vi "ADMIN -Process Customize for Company.vi"(0 "SET":T2=enum."GET ALL", 2 "CfgValues":string[][](array[string])=[["", ""], ["CompanyName", "ABC Test Labs Inc"], ["LogoFileName", "ABC.png"], ["CSACategory", "II"], ["HomeAddrLine00", "McIntosh Lalani Engineering LTD."], ["HomeAddrLine01", "Bay 10,4604 - 13th Street NE"], ["HomeAddLine02", "Calgary AB  T2E 6P1"], ["HomeAddrLine03", "CANADA"], ["", ""], ["DeltaTestTime", "120"], ["", ""], ["PDFRptDir", "C:\\Program Files (x86)\\BreakTest\\PDF_ARCHIVE"], ["PDFRes", "8-Bit Gray Scale"], ["PDFDrvName", "Black Ice PDF"], ["PDFAlertDays", "2"], ["WebPortalURL", "-"], ["", ""], ["DshBrdEnabled", "Yes"], ["DshBrdEvntNeedsAction", "Yes"], ["DshBrdEvntNew", "Yes"], ["DshBrdEvntUpdate", "Yes"], ["DshBrdEvntSignature", "Yes"], ["DshBrdEvntAgeData", "Yes"], ["", ""], ["EmailSvrAddr", "shawmail.cg.shawcable.net"], ["EmailAddr", "emmanual@shaw.ca"], ["EmailAccName", "Immanuel Nwachukwu"], ["EmailSize", "5"], ["", ""], ["FTPDir", "-"], ["FTPAddr", "ftp.mezintel.com"], ["FTPUser", "breaktestrpts@mezintel.com"], ["FTPPswd", "Break123"], ["", ""], ["UtilStartDate", "2011/09/26"], ["GSTPercent", "5"], ["CostPerTest", "1.5"], ["VendorAddrLine00", "Mezintel Inc."], ["VendorAddrLine01", "20 Citadel Hills Green NW"], ["VendorAddrLine02", "Calgary, AB, T3G 3T5"], ["VendorAddrLine03", "CANADA"]], 3 "KEY":string, 5 "error in (no error)":errorcluster, 8 "path to PNG file":path) -> (13 "Found":bool, 14 "ALL -Out":T1={"CurrPath"=path "C:/MEZINTEL PROJECTS/PERFORCE MEZINTEL PROJECTS/BreakTest 3/BreakTest Source/SOURCE CODE", "LogoPic"=bytes[30000], "LogoPicRed"=bytes[2727], "CoName"="ABC Test Labs Inc", "CSACategory"="II", "Home CoID|DivID"=["47", "52"], "ParmKey|Value"=[["LogoFileName", "ABC.png"], ["CompanyName", "ABC Test Labs Inc"], ["CSACategory", "II"], ["PDFRptDir", "C:\\Program Files (x86)\\BreakTest\\PDF_ARCHIVE"], ["PDFRes", "8-Bit Gray Scale"], ["DshBrdEnabled", "Yes"], ["EmailSvrAddr", "shawmail.cg.shawcable.net"], ["EmailAddr", "emmanual@shaw.ca"], ["EmailAccName", "Immanuel Nwachukwu"], ["EmailSize", "5"], ["PDFDrvName", "Black Ice PDF"], ["PDFAlertDays", "2"], ["FTPAddr", "ftp.mezintel.com"], ["FTPUser", "breaktestrpts@mezintel.com"], ["FTPPswd", "Break123"], ["WebPortalURL", "-"]], "PicRef"=refnum, "DBParmKey|Value"=[]}, 15 "VALUE":string, 18 "ClrRes":i32, 19 "error out":errorcluster)   [LabVIEW 2019]
uses:
  ctlFNCoCustomization.ctl
  ctlADMIN-CoCfgParamsOut.ctl
  <vilib>/Utility/config.llb/Read Key (String).vi
  <vilib>/Utility/config.llb/Write Key (String).vi
  <vilib>/Utility/config.llb/NI_LVConfig.lvlib
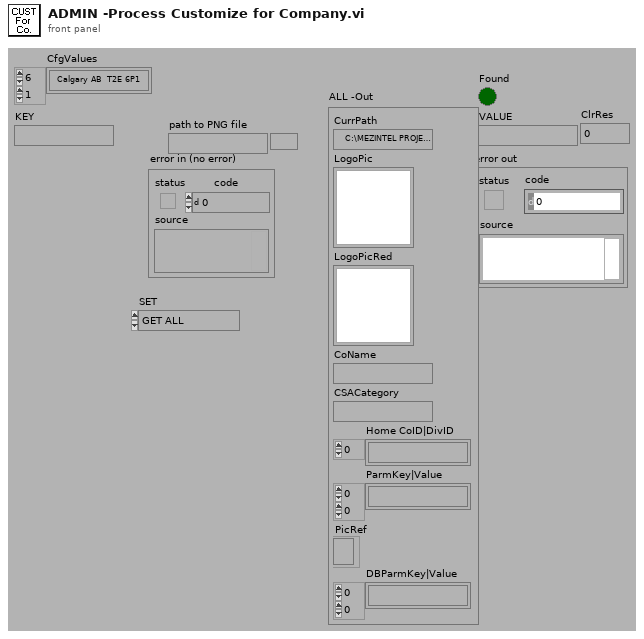
[diagram p1: front panel]
types:
  T1 = typedef "ctlADMIN-CoCfgParamsOut.ctl" = cluster{"CurrPath":path, "LogoPic":picture, "LogoPicRed":picture, "CoName":string, "CSACategory":string, "Home CoID|DivID":string[], "ParmKey|Value":string[][], "PicRef":refnum<k7>, "DBParmKey|Value":string[][]}
  T2 = typedef "ctlFNCoCustomization.ctl" = enum16{"pre-init", "Init", "Write Co. Info to ini", "GET CFG PARAM", "GET Param Value for Name", "GET ALL"}
  T3 = cluster{"path to PNG file":path, "LogoPic":picture, "LogoPicRed":picture, "CoName":string, "CSACategory":string, "Home CoID|DivID":string[], "ParmKey|Value":string[][], "PicRef":refnum<k7>, "DBParmKey|Value":string[][]}
  T4 = typedef "NI_LVConfig.lvlib/Config Data RefNum.ctl" = refnum<k1>
  T5 = typedef "imagedata.ctl" = cluster{"image type":i32, "image depth":i32, "image":u8[], "mask":u8[], "colors":u32[], "Rectangle":cluster{"left":i16, "top":i16, "right":i16, "bottom":i16}}
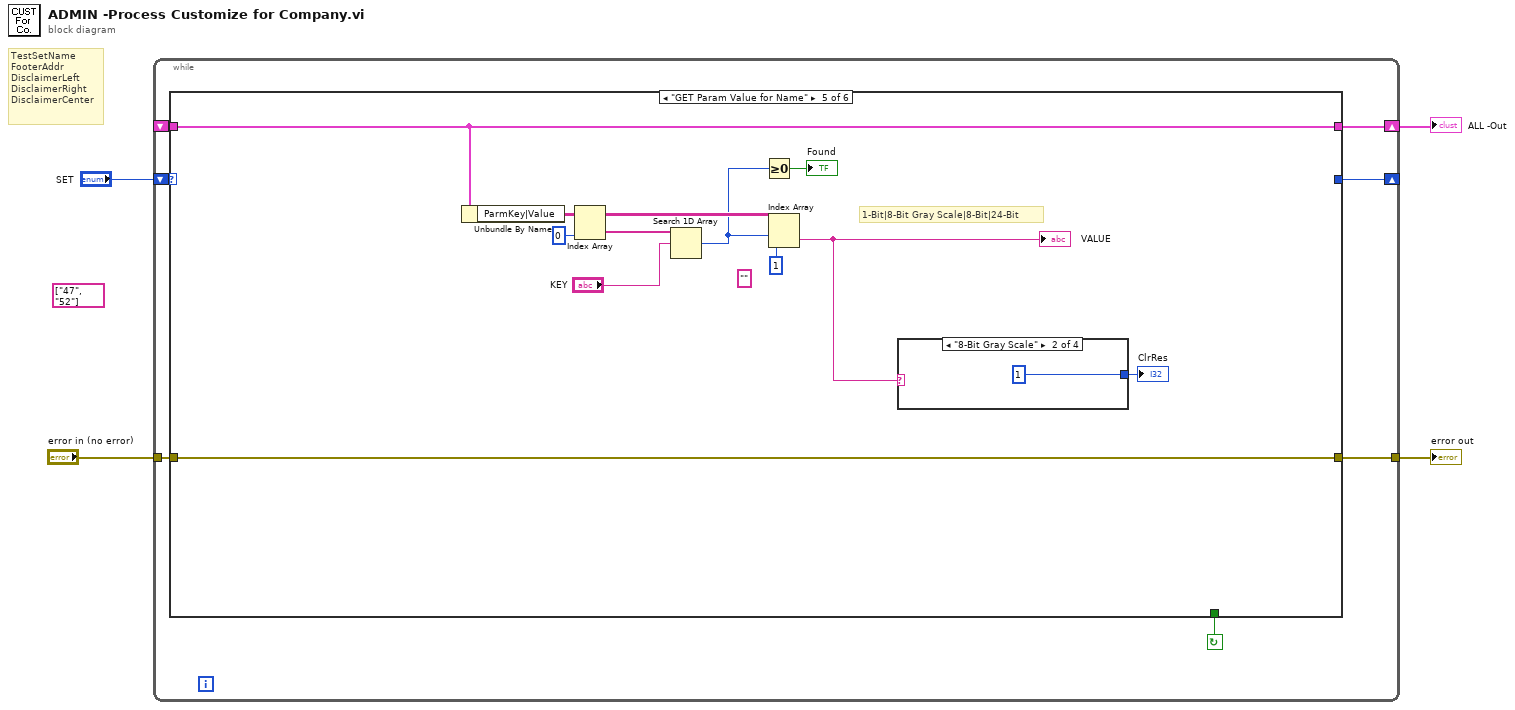
[diagram p0: block diagram]
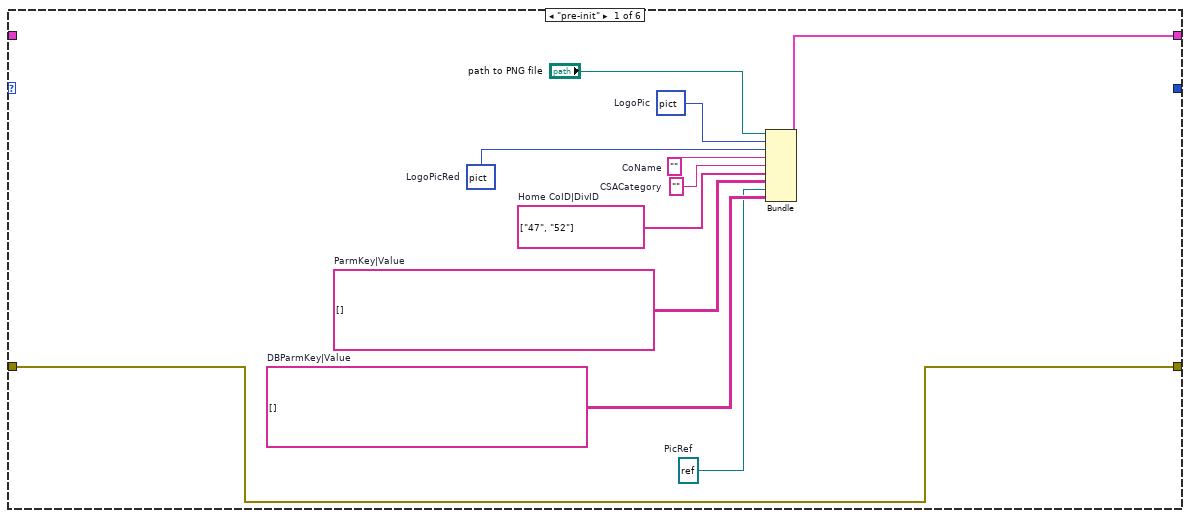
[diagram p2: hidden frame]
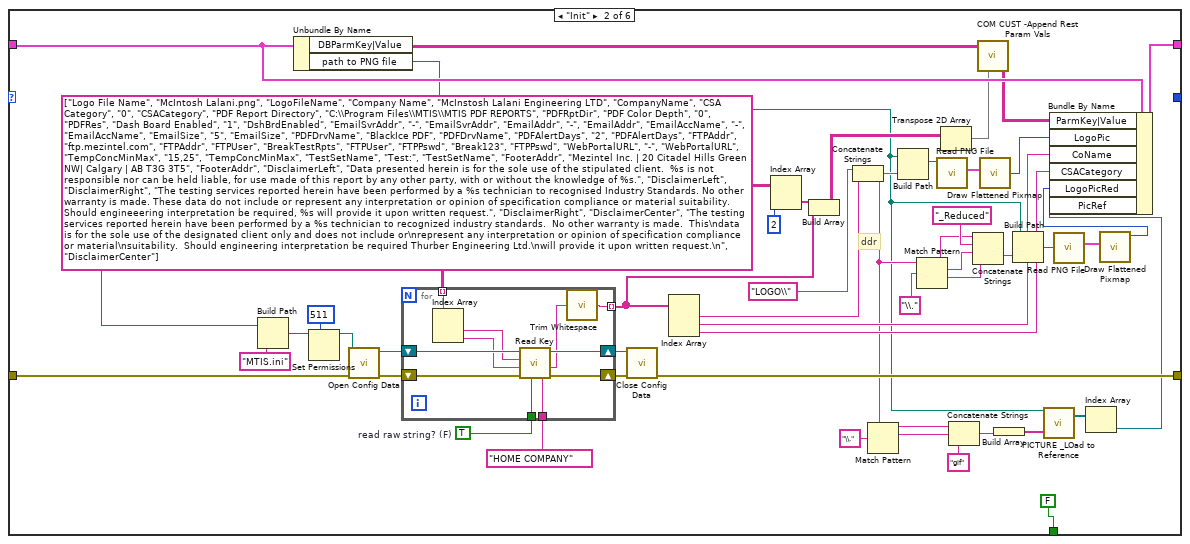
[diagram p3: hidden frame]
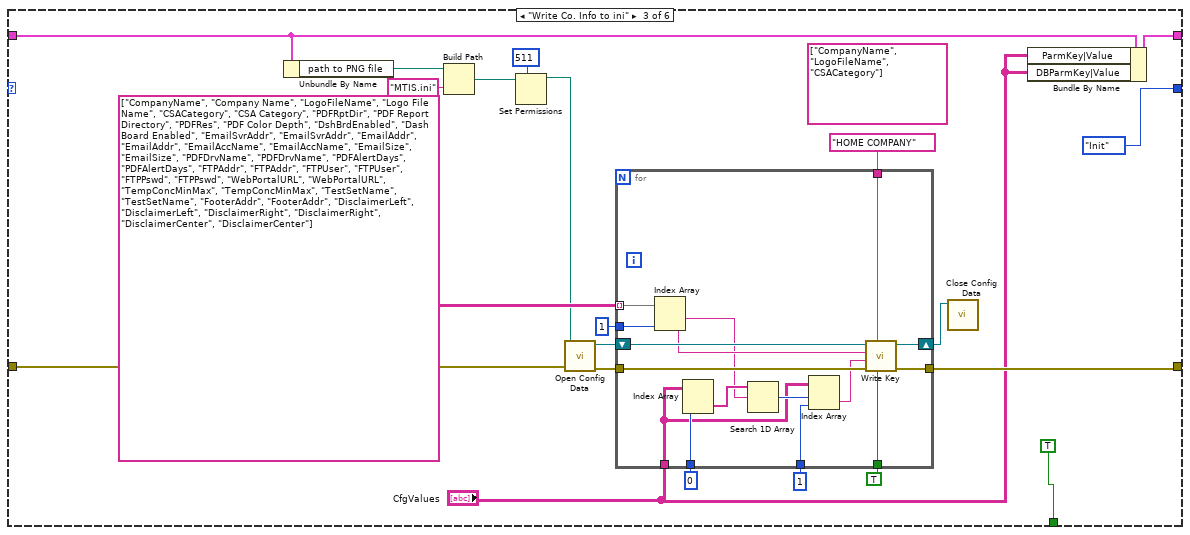
[diagram p4: hidden frame]
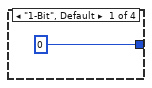
[diagram p6: hidden frame]
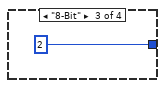
[diagram p7: hidden frame]
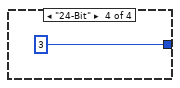
[diagram p8: hidden frame]
diagram:
  (unwired) string[] ["47", "52"] ("Home CoID|DivID")
  # "TestSetName\nFooterAddr\nDisclaimerLeft\nDisclaimerRight\nDisclaimerCenter"
  n1 = while {
    tunnel: [w10] -> w3
    tunnel: "error in (no error)" -> [w9]
    shift-right: [w6] -> w1
    shift-left: _ -> [w7]
    shift-right: [w5] -> _
    shift-left: "SET" -> [w11]
    stop <- w8 continue-if-true
    n2 = case shown="\"GET Param Value for Name\"" w11 {
      tunnel: [w13 w67 w84 w121 w132 w138] -> w10
      tunnel: w9 -> [w13 w66 w102 w121 w132 w138]
      tunnel: [_ FALSE TRUE _ _ _] -> w8
      tunnel: w7 -> [_ w52 w92 w120 w131 w137]
      tunnel: [w14 w57 w91 w120 w131 w137] -> w6
      tunnel: [_ _ ctlFNCoCustomization."Init" ("SET") _ _ _] -> w5
      frame "pre-init" {
        w22 = string[][] []  # DBParmKey|Value
        w21 = refnum<k7> refnum  # PicRef
        w20 = picture data[5B]  # LogoPicRed
        w19 = string[][] []  # ParmKey|Value
        w18 = string[] ["47", "52"]  # Home CoID|DivID
        w15 = picture data[5B]  # LogoPic
        w17 = ""  # CSACategory
        w16 = ""  # CoName
        n3 = Bundle("path to PNG file"="path to PNG file", "LogoPic"=w15, "LogoPicRed"=w20, "CoName"=w16, "CSACategory"=w17, "Home CoID|DivID"=w18, "ParmKey|Value"=w19, "PicRef"=w21, "DBParmKey|Value"=w22) -> (w14:T3)  [unwired: 1 out]
      }
      frame "Init" {
        w33 = string[][] [["Logo File Name", "McIntosh Lalani.png", "LogoFileName"], ["Company Name", "McInstosh Lalani Engineering LTD", "CompanyName"], ["CSA Category", "0", "CSACategory"], ["PDF Report Directory", "C:\\Program Files\\MTIS\\MTIS PDF REPORTS", "PDFRptDir"], ["PDF Color Depth", "0", "PDFRes"], ["Dash Board Enabled", "1", "DshBrdEnabled"], ["EmailSvrAddr", "-", "EmailSvrAddr"], ["EmailAddr", "-", "EmailAddr"], ["EmailAccName", "-", "EmailAccName"], ["EmailSize", "5", "EmailSize"], ["PDFDrvName", "BlackIce PDF", "PDFDrvName"], ["PDFAlertDays", "2", "PDFAlertDays"], ["FTPAddr", "ftp.mezintel.com", "FTPAddr"], ["FTPUser", "BreakTestRpts", "FTPUser"], ["FTPPswd", "Break123", "FTPPswd"], ["WebPortalURL", "-", "WebPortalURL"], ["TempConcMinMax", "15,25", "TempConcMinMax"], ["TestSetName", "Test:", "TestSetName"], ["FooterAddr", "Mezintel Inc. | 20 Citadel Hills Green NW| Calgary | AB T3G 3T5", "FooterAddr"], ["DisclaimerLeft", "Data presented herein is for the sole use of the stipulated client.  %s is not responsible nor can be held liable, for use made of this report by any other party, with or without the knowledge of %s.", "DisclaimerLeft"], ["DisclaimerRight", "The testing services reported herein have been performed by a %s technician to recognised Industry Standards. No other warranty is made. These data do not include or represent any interpretation or opinion of specification compliance or material suitability. Should engineeering interpretation be required, %s will provide it upon written request.", "DisclaimerRight"], ["DisclaimerCenter", "The testing services reported herein have been performed by a %s technician to recognized industry standards.  No other warranty is made.  This\ndata is for the sole use of the designated client only and does not include or\nrepresent any interpretation or opinion of specification compliance or material\nsuitability.  Should engineering interpretation be required Thurber Engineering Ltd.\nwill provide it upon written request.\n", "DisclaimerCenter"]]
        w61 = TRUE  # read raw string? (F)
        # "ddr"
        n4 = Unbundle By Name(w52) -> ("DBParmKey|Value"=w26:string[][], "path to PNG file"=w23:path)
        n5 = Build Path(base path=w23, name or relative path="MTIS.ini") -> (appended path=w63:path)
        n6 = Set Permissions(7:i16 511 ("permissions"), 11:w63) -> (3:w28:path)  [unwired: 1 in, 3 out]
        n7 = call <vilib>:"Open Config Data.vi"("error in (no error)"=w66, "configuration file path"=w28) -> ("error out"=w65:errorcluster, "refnum"=w62:T4)  [unwired: 7 in, 1 out]
        n8 = for {
          shift-right: [w79] -> w60
          shift-left: w62 -> [w80]
          tunnel: w33 -> [w78] mode=indexing
          tunnel: w61 -> [w75]
          shift-right: [w81] -> w64
          shift-left: w65 -> [w82]
          tunnel: [w72] -> w29 mode=indexing
          tunnel: "HOME COMPANY" ("section") -> [w73]
          n9 = Index Array(array=w78) -> (element #1=w77:string, element #2=w76:string)  [unwired: 2 in]
          n10 = call-poly <vilib>:"Read Key.vi"("read raw string? (F)"=w75, "section"=w73, "error in (no error)"=w82, "default value"=w76, "key"=w77, "refnum"=w80) -> ("error out"=w81:errorcluster, "value"=w74:string, "refnum out"=w79:T4)  [unwired: 3 out]
          n11 = call <vilib>:"Trim Whitespace.vi"("string"=w74) -> ("trimmed string"=w72:string)  [unwired: 1 in]
        }
        n12 = call <vilib>:"Close Config Data.vi"("error in (no error)"=w64, "refnum"=w60) -> ("error out"=w67:errorcluster)  [unwired: 1 in, 8 out]
        n13 = Index Array(array=w29) -> (element #1=w59:string, element #2=w55:string, element #3=w54:string)  [unwired: 3 in]
        n14 = Index Array(array=w33, index (col)=2 ("disabled index (col)")) -> (element=w31:string[])  [unwired: 1 in]
        n15 = Build Array(w31, w29) -> (w30:string[][])
        n16 = Concatenate Strings("LOGO\\" ("string"), w59) -> (w42:string)
        n17 = Match Pattern(string=w42, regular expression="\\.") -> (before substring=w40:string, match substring=w39:string)  [unwired: 3 out]
        n18 = Build Path(base path=w23, name or relative path=w42) -> (appended path=w70:path)
        n19 = Match Pattern(string=w42, regular expression="\\.") -> (before substring=w47:string, match substring=w49:string, after substring=w50:string)  [unwired: 2 out]
        n20 = call <vilib>:"Read PNG File.vi"("path to PNG file"=w70) -> ("image data"=w69:T5)  [unwired: 1 in, 9 out]
        n21 = Transpose 2D Array(2D array=w30) -> (transposed array=w25:string[][])
        n22 = Concatenate Strings(w40, w39, "gif" ("string")) -> (w34:string)
        n23 = Concatenate Strings(w47, "_Reduced" ("string"), w49, w50) -> (w46:string)
        n24 = call "COM CUST -Append Rest Param Vals.vi"("DBParmKey|Value"=w26, "LclParamVal"=w25) -> ("AllParamvalue"=w24:string[][])  [unwired: 17 out]
        n25 = call <vilib>:"Draw Flattened Pixmap.vi"("image data"=w69) -> ("new picture"=w56:picture)  [unwired: 1 in, 7 out]
        n26 = Build Array(w34) -> (w37:string[])
        n27 = Build Path(base path=w23, name or relative path=w46) -> (appended path=w44:path)
        n28 = call "PICTURE _LOad to Reference.vi"("Path"=w23, "ImagePaths"=w37) -> ("PicRefs"=w36:refnum<k7>[])  [unwired: 1 in, 16 out]
        n29 = call <vilib>:"Read PNG File.vi"("path to PNG file"=w44) -> ("image data"=w45:T5)  [unwired: 1 in, 9 out]
        n30 = Index Array(array=w36) -> (element=w35:refnum<k7>)  [unwired: 1 in]
        n31 = call <vilib>:"Draw Flattened Pixmap.vi"("image data"=w45) -> ("new picture"=w43:picture)  [unwired: 1 in, 7 out]
        n32 = Bundle By Name(cluster=w52, "ParmKey|Value"=w24, "LogoPic"=w56, "CoName"=w55, "CSACategory"=w54, "LogoPicRed"=w43, "PicRef"=w35) -> (w57:T3)
      }
      frame "Write Co. Info to ini" {
        (unwired) string[] ["CompanyName", "LogoFileName", "CSACategory"]
        n33 = Unbundle By Name(w92) -> ("path to PNG file"=w95:path)
        n34 = Build Path(base path=w95, name or relative path="MTIS.ini") -> (appended path=w87:path)
        n35 = Set Permissions(7:i16 511 ("permissions"), 11:w87) -> (3:w86:path)  [unwired: 1 in, 3 out]
        n36 = call <vilib>:"Open Config Data.vi"("error in (no error)"=w102, "configuration file path"=w86) -> ("error out"=w101:errorcluster, "refnum"=w100:T4)  [unwired: 7 in, 1 out]
        n37 = for {
          tunnel: "HOME COMPANY" ("section") -> [w115]
          shift-right: [w116] -> w99
          shift-left: w100 -> [w117]
          tunnel: w101 -> [w119]
          tunnel: [w118] -> w84
          tunnel: string[][] [["CompanyName", "Company Name"], ["LogoFileName", "Logo File Name"], ["CSACategory", "CSA Category"], ["PDFRptDir", "PDF Report Directory"], ["PDFRes", "PDF Color Depth"], ["DshBrdEnabled", "Dash Board Enabled"], ["EmailSvrAddr", "EmailSvrAddr"], ["EmailAddr", "EmailAddr"], ["EmailAccName", "EmailAccName"], ["EmailSize", "EmailSize"], ["PDFDrvName", "PDFDrvName"], ["PDFAlertDays", "PDFAlertDays"], ["FTPAddr", "FTPAddr"], ["FTPUser", "FTPUser"], ["FTPPswd", "FTPPswd"], ["WebPortalURL", "WebPortalURL"], ["TempConcMinMax", "TempConcMinMax"], ["TestSetName", "TestSetName"], ["FooterAddr", "FooterAddr"], ["DisclaimerLeft", "DisclaimerLeft"], ["DisclaimerRight", "DisclaimerRight"], ["DisclaimerCenter", "DisclaimerCenter"]] -> [w114] mode=indexing
          tunnel: "CfgValues" -> [w107]
          tunnel: 1 ("index") -> [w111]
          tunnel: 0 ("disabled index (col)") -> [w113]
          tunnel: 1 ("disabled index (col)") -> [w106]
          tunnel: TRUE ("write raw string? (F)") -> [w104]
          n38 = Index Array(array=w114, index #2=w111) -> (element #1=w109:string, element #2=w110:string)  [unwired: 1 in]
          n39 = Index Array(array=w107, index (col)=w113) -> (element=w112:string[])  [unwired: 1 in]
          n40 = Search 1D Array(1D array=w112, element=w109) -> (index of element=w108:i32)  [unwired: 1 out]
          n41 = Index Array(array=w107, index (row)=w108, index (col)=w106) -> (element=w105:string)
          n42 = call-poly <vilib>:"Write Key.vi"("write raw string? (F)"=w104, "section"=w115, "error in (no error)"=w119, "value"=w105, "key"=w110, "refnum"=w117) -> ("error out"=w118:errorcluster, "refnum out"=w116:T4)  [unwired: 4 out]
        }
        n43 = call <vilib>:"Close Config Data.vi"("refnum"=w99) -> ()  [unwired: 2 in, 9 out]
        n44 = Bundle By Name(cluster=w92, "ParmKey|Value"="CfgValues", "DBParmKey|Value"="CfgValues") -> (w91:T3)
      }
      frame "GET CFG PARAM" {
      }
      frame "GET Param Value for Name" {
        (unwired) "" ("element")
        # "1-Bit|8-Bit Gray Scale|8-Bit|24-Bit"
        n45 = Unbundle By Name(w131) -> ("ParmKey|Value"=w127:string[][])
        n46 = Index Array(array=w127, index (col)=0 ("disabled index (col)")) -> (element=w130:string[])  [unwired: 1 in]
        n47 = Search 1D Array(1D array=w130, element="KEY") -> (index of element=w126:i32)  [unwired: 1 out]
        n48 = Greater Or Equal To 0?(x=w126) -> (x >= 0?=→"Found":bool)
        n49 = Index Array(array=w127, index (row)=w126, index (col)=1 ("disabled index (col)")) -> (element=w124:string)
        "VALUE" <- w124
        n50 = case shown="\"8-Bit Gray Scale\"" w124 {
          tunnel: [0 1 2 3] -> w123
          frame "1-Bit", Default {
          }
          frame "8-Bit Gray Scale" {
          }
          frame "8-Bit" {
          }
          frame "24-Bit" {
          }
        }
        "ClrRes" <- w123
      }
      frame "GET ALL" {
      }
    }
  }
  "error out" <- w3
  "ALL -Out" <- w1
